vi "AerotechSetTarget.vi"(0 "error in (no error)":errorcluster, 5 "AEROTECH.TARGET":T1) -> (3 "error out":errorcluster)   [LabVIEW 2009]
uses:
  Controls/AerotechTarget.ctl
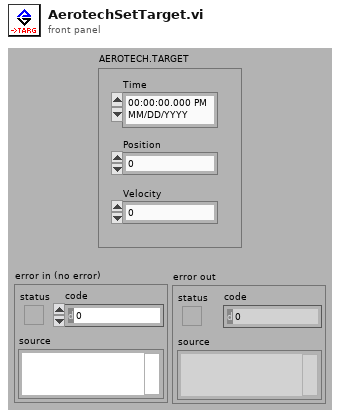
[diagram p1: front panel]
types:
  T1 = typedef "AerotechTarget.ctl" = cluster{"Time":timestamp, "Position":dbl, "Velocity":dbl}
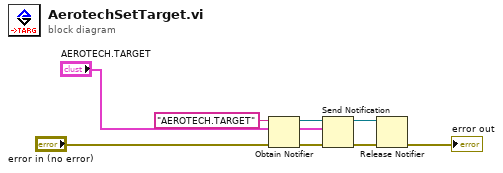
[diagram p0: block diagram]
diagram:
  n1 = Obtain Notifier(name (unnamed)="AEROTECH.TARGET", notification data type="AEROTECH.TARGET", error in (no error)="error in (no error)") -> (notifier out=w6:refnum<notifier>, error out=w7:errorcluster)  [unwired: 1 in, 1 out]
  n2 = Send Notification(notification="AEROTECH.TARGET", notifier=w6, error in (no error)=w7) -> (notifier out=w3:refnum<notifier>, error out=w4:errorcluster)
  n3 = Release Notifier(notifier=w3, error in (no error)=w4) -> (error out=→"error out":errorcluster)  [unwired: 1 in, 2 out]
